vi "naked test.vi"() -> ()   [LabVIEW 2023]
uses:
  <instrlib>/niScope/Controls/niScope vertical coupling.ctl
  <instrlib>/niScope/Controls/niScope timestamp type.ctl
  <instrlib>/niScope/Configure/Trigger/niScope Configure Trigger Immediate.vi
  <instrlib>/niScope/Acquire/Fetch/niScope Fetch WDT.vi
panel:
  out "acquisition status 3":i32 caption="acquisition status"
  out "acquisition status 2":i32 caption="acquisition status0"
  out "acquisition status":i32 caption="acquisition status1"
  out "Waveform From Scope":waveform(dbl)(graph) caption="Waveform from Scope"
  in  "Stop":bool caption="stop"
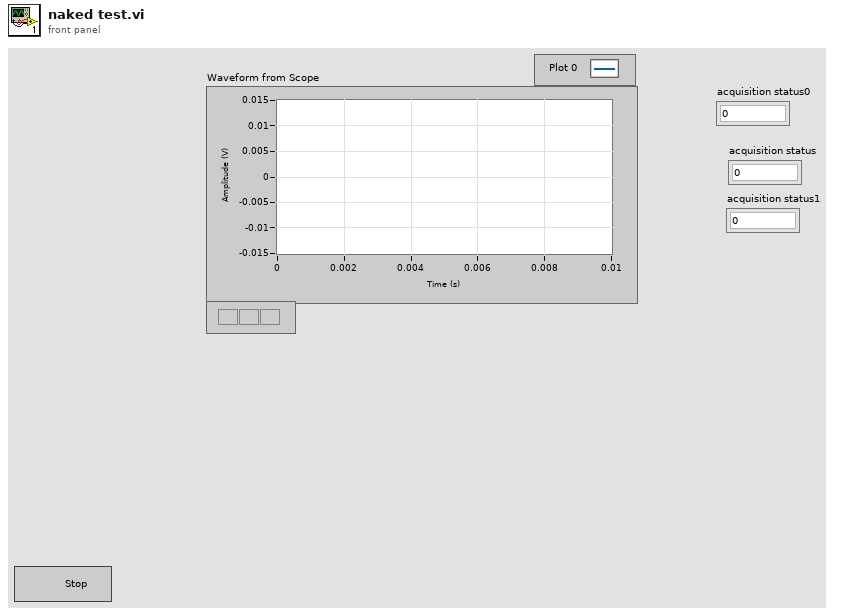
[diagram p1: front panel]
types:
  T1 = typedef "niScope timestamp type.ctl" = i32
  T2 = typedef "niScope vertical coupling.ctl" = i32
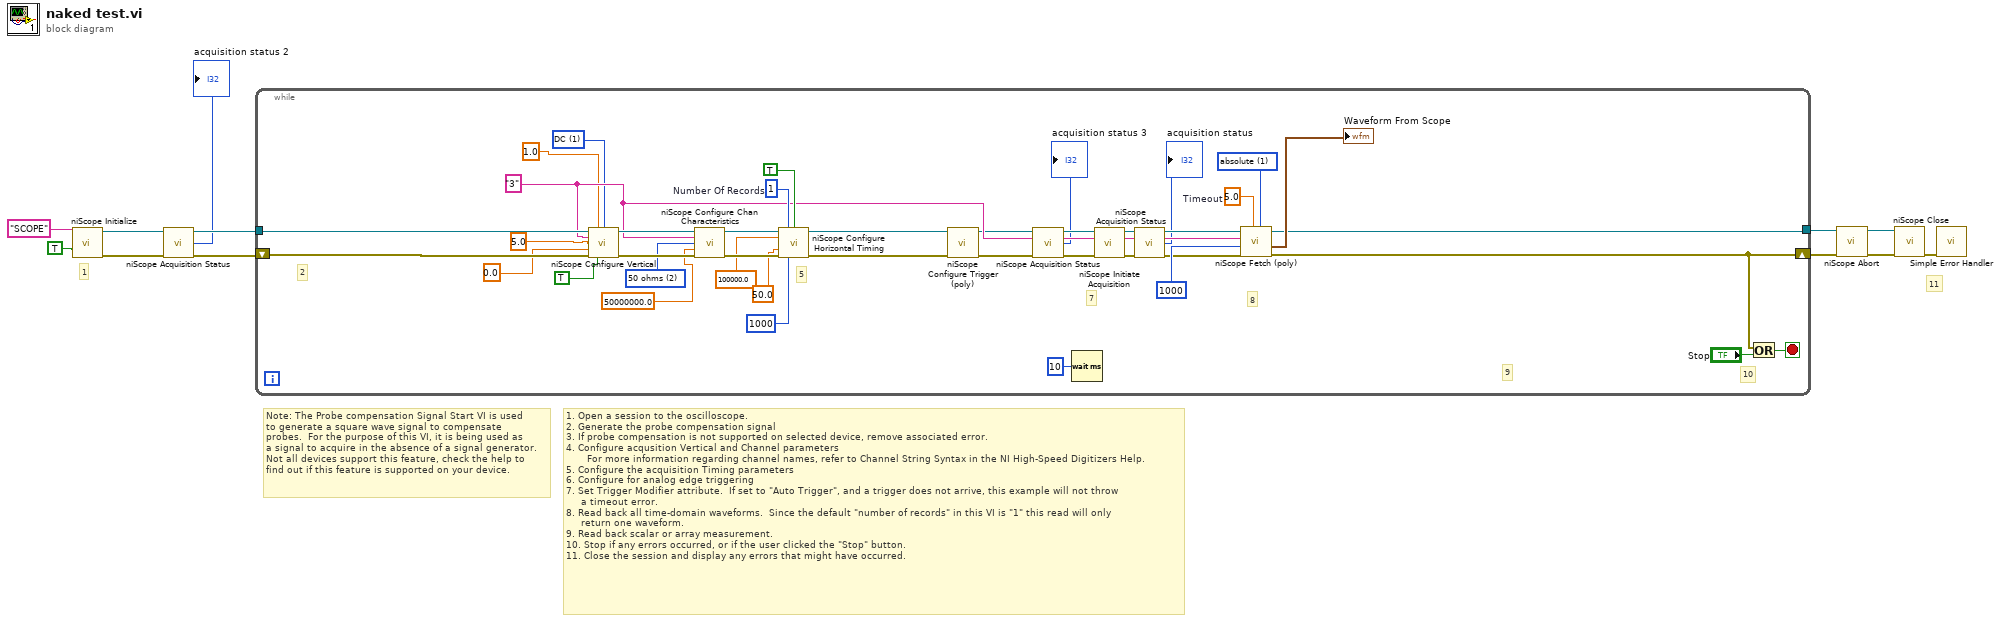
[diagram p0: block diagram]
diagram:
  # "Note: The Probe compensation Signal Start VI is used\nto generate a square wave signal to compensate\nprobes.  For the purpose of this VI, it is being used as\na signal to acquire in the absence of a signal generator.\nNot all devices support this feature, check the help to\nfind out if this feature is supported on your device."
  # "11"
  # "1"
  # "1. Open a session to the oscilloscope.\n2. Generate the probe compensation signal \n3. If probe compensation is not supported on selected device, remove associated error.\n4. Configure acqusition Vertical and Channel parameters\n       For more information regarding channel names, refer to Channel String Syntax in the NI High-Speed Digitizers Help.\n5. Configure the acquisition Timing parameters\n6. Configure for analog edge triggering\n7. Set Trigger Modifier attribute.  If set to \"Auto Trigger\", and a trigger does not arrive, this example will not throw\n     a timeout error.\n8. Read back all time-domain waveforms.  Since the default \"number of records\" in this VI is \"1\" this read will only\n     return one waveform.\n9. Read back scalar or array measurement.\n10. Stop if any errors occurred, or if the user clicked the \"Stop\" button.\n11. Close the session and display any errors that might have occurred."
  n1 = call <instrlib>:"niScope Initialize.vi"("resource name"="SCOPE", "reset device"=TRUE) -> ("instrument handle"=w3:refnum<k15>, "error out"=w11:errorcluster)  [unwired: 12 in]
  n2 = call <instrlib>:"niScope Acquisition Status.vi"("instrument handle"=w3, "error in"=w11) -> ("instrument handle out"=w2:refnum<k15>, "acquisition status"=→"acquisition status 2":i32, "error out"=w4:errorcluster)  [unwired: 11 in]
  n3 = while {
    tunnel: w2 -> [w41]
    tunnel: [w46] -> w7
    shift-right: [w45] -> w10
    shift-left: w4 -> [w44]
    stop <- w51 stop-if-true
    w21 = T1 1 items=["relative", "absolute"] ("timestamp Type")
    w28 = u32 2 items=["1 mega ohm"=0, "50 ohms"=2] ("input impedance")
    w31 = T2 1 items=["AC", "DC", "Ground"] ("vertical coupling")
    w32 = "3" ("channels")
    w36 = 1  # Number Of Records
    w42 = 5.0  # Timeout
    # "9"
    # "8"
    # "5"
    # "2"
    # "10"
    # "7"
    n4 = call <instrlib>:"niScope Configure Vertical.vi"("instrument handle"=w41, "probe attenuation"=1.0, "vertical coupling"=w31, "channels"=w32, "vertical range"=5.0, "vertical offset"=0.0, "error in"=w44, "channel enabled"=TRUE) -> ("instrument handle out"=w39:refnum<k15>, "error out"=w40:errorcluster)  [unwired: 6 in]
    n5 = call <instrlib>:"niScope Configure Chan Characteristics.vi"("instrument handle"=w39, "channels"=w32, "input impedance"=w28, "maximum input frequency"=50000000.0, "error in"=w40) -> ("instrument handle out"=w38:refnum<k15>, "error out"=w37:errorcluster)  [unwired: 9 in]
    n6 = call <instrlib>:"niScope Configure Horizontal Timing.vi"("instrument handle"=w38, "number of records"=w36, "enforce realtime"=TRUE ("Enforce Realtime"), "min sample rate"=100000.0, "reference position"=50.0, "error in"=w37, "min record length"=1000) -> ("instrument handle out"=w47:refnum<k15>, "error out"=w48:errorcluster)  [unwired: 7 in]
    n7 = call-poly <instrlib>:"niScope Configure Trigger (poly).vi"("instrument handle"=w47, "error in"=w48) -> ("instrument handle out"=w15:refnum<k15>, "error out"=w43:errorcluster)  [unwired: 12 in]
    n8 = call <instrlib>:"niScope Acquisition Status.vi"("instrument handle"=w15, "error in"=w43) -> ("instrument handle out"=w14:refnum<k15>, "acquisition status"=→"acquisition status 3":i32, "error out"=w16:errorcluster)  [unwired: 11 in]
    n9 = Wait (ms)(milliseconds to wait=u32 10 ("Millisecond Multiple")) -> ()  [unwired: 1 out]
    n10 = call <instrlib>:"niScope Initiate Acquisition.vi"("instrument handle"=w14, "error in"=w16) -> ("instrument handle out"=w19:refnum<k15>, "error out"=w22:errorcluster)  [unwired: 12 in]
    n11 = call <instrlib>:"niScope Acquisition Status.vi"("instrument handle"=w19, "error in"=w22) -> ("instrument handle out"=w18:refnum<k15>, "acquisition status"=→"acquisition status":i32, "error out"=w20:errorcluster)  [unwired: 11 in]
    n12 = call-poly <instrlib>:"niScope Fetch (poly).vi"("timestamp Type"=w21, "timeout"=w42, "error in"=w20, "numSamples"=1000, "channels"=w32, "instrument handle"=w18) -> ("error out"=w45:errorcluster, "wfm"=→"Waveform From Scope":waveform(dbl), "instrument handle out"=w46:refnum<k15>)  [unwired: 2 in, 1 out]
    n13 = Or(x=w45, y="Stop") -> (x .or. y?=w51:bool)
  }
  n14 = call <instrlib>:"niScope Abort.vi"("instrument handle"=w7, "error in"=w10) -> ("instrument handle out"=w6:refnum<k15>, "error out"=w8:errorcluster)  [unwired: 12 in]
  n15 = call <instrlib>:"niScope Close.vi"("instrument handle"=w6, "error in"=w8) -> ("error out"=w12:errorcluster)  [unwired: 13 in]
  n16 = call <vilib>:"Simple Error Handler.vi"("error in (no error)"=w12) -> ()  [unwired: 4 in, 5 out]
